vi "C4Ftr_getAccsessMode.vi"(0 "c4Ftr in":refnum<k24>, 11 "error in":errorcluster) -> (4 "c4Ftr out":refnum<k24>, 6 "accessMode out":i64(ring) items=["UNKNOWN", "NI", "NA", "RO", "WO", "RW"], 15 "error out":errorcluster)   [LabVIEW 2015, in "libC4HdlLV.lvlib"]
uses:
  libC4HdlLV.lvlib
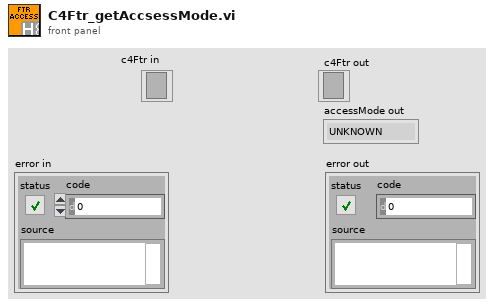
[diagram p1: front panel]
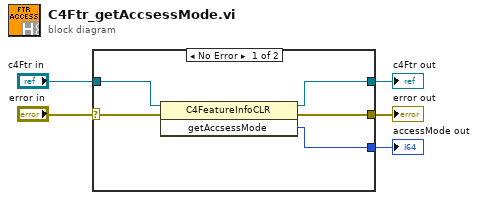
[diagram p0: block diagram]
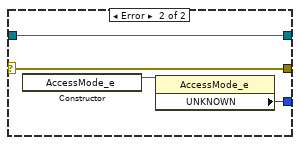
[diagram p2: hidden frame]
diagram:
  n1 = case shown="No Error" "error in" {
    selector: "error in" -> [w10 w14]
    tunnel: "c4Ftr in" -> [w9 w13]
    tunnel: [w8 w11] -> w1
    tunnel: [w7 w14] -> w3
    tunnel: [w6 w13] -> w2
    frame No Error {
      n2 = invoke class="C4FeatureInfoCLR" method="getAccsessMode"(reference=w9, error in=w10) -> (reference out=w6:refnum<k24>, error out=w7:errorcluster, "getAccsessMode"=w8:i64)  [unwired: 1 in]
    }
    frame Error {
      n3 = constructor class="AccessMode_e"() -> (reference out=w12:refnum<k24>)  [unwired: 3 in, 2 out]
      n4 = property class="AccessMode_e"(reference=w12) -> ("UNKNOWN"=w11:i64)  [unwired: 1 in, 2 out]
    }
  }
  "error out" <- w3
  "c4Ftr out" <- w2
  "accessMode out" <- w1
